vi "GLdrv_FILE_TRANS_SIZE.vi"(0 "Connection ID":T1, 11 "error in (no error)":errorcluster) -> (4 "Connection ID Out":T1, 6 "Size out":dbl, 15 "error out":errorcluster)   [LabVIEW 2017, in "GL860_Driver.lvlib"]
doc: "記録計本体内のファイルを転送します\nファイルサイズ（バイト数）の参照\nSOURceで設定したファイルのバイト数を参照します\n例）　；FILE:TRANS:SIZE 12345　（12345Byte)"
uses:
  GL860_Driver.lvlib
  ConnectionID.ctl
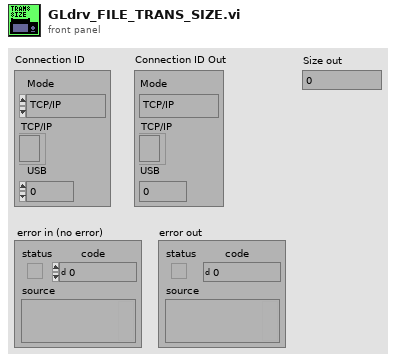
[diagram p1: front panel]
types:
  T1 = typedef "ConnectionID.ctl" = cluster{"Mode":enum16{"TCP/IP", "USB"}, "TCP/IP":refnum<k5>, "USB":i32}
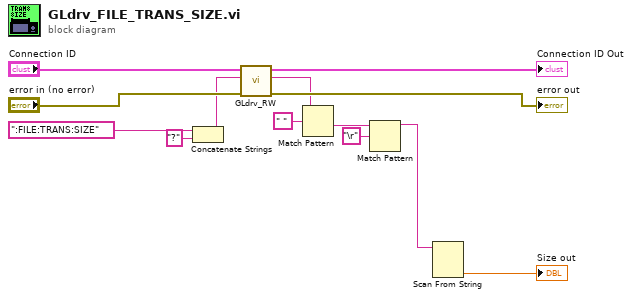
[diagram p0: block diagram]
diagram:
  n1 = Concatenate Strings(":FILE:TRANS:SIZE" ("Command"), "?" ("string")) -> (w2:string)
  n2 = call "GLdrv_RW.vi"("error in (no error)"="error in (no error)", "data in"=w2, "Connection ID"="Connection ID") -> ("error out"=→"error out":errorcluster, "data out"=w1:string, "Connection ID Out"=→"Connection ID Out":T1)  [unwired: 4 in, 2 out]
  n3 = Match Pattern(string=w1, regular expression=" " ("search string/char (-)")) -> (after substring=w5:string)  [unwired: 4 out]
  n4 = Match Pattern(string=w5, regular expression="\r") -> (before substring=w3:string)  [unwired: 4 out]
  n5 = Scan From String(input string=w3) -> (output 1=→"Size out":dbl)  [unwired: 3 in, 4 out]
